vi "TFTP Get File.vi"(5 "net address":string, 6 "Binary (T)":bool=TRUE, 7 "timeout ms (1000)":i32=1000, 8 "error in (no error)":errorcluster, 9 "local path":path, 10 "remote path":string, 11 "Host":string) -> (0 "error out":errorcluster, 2 "file error":errorcluster, 3 "File Length":i32)   [LabVIEW 2016]
doc: "Connects to an TFTP server and copies a single file to the local machine."
panel:
  out "local port":u16
  out "server port":u16
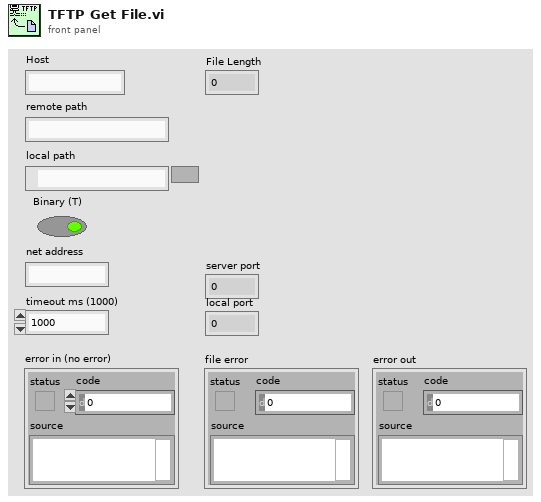
[diagram p1: front panel]
types:
  T1 = enum16{"open", "replace", "create", "open or create", "replace or create", "replace or create with confirmation"}
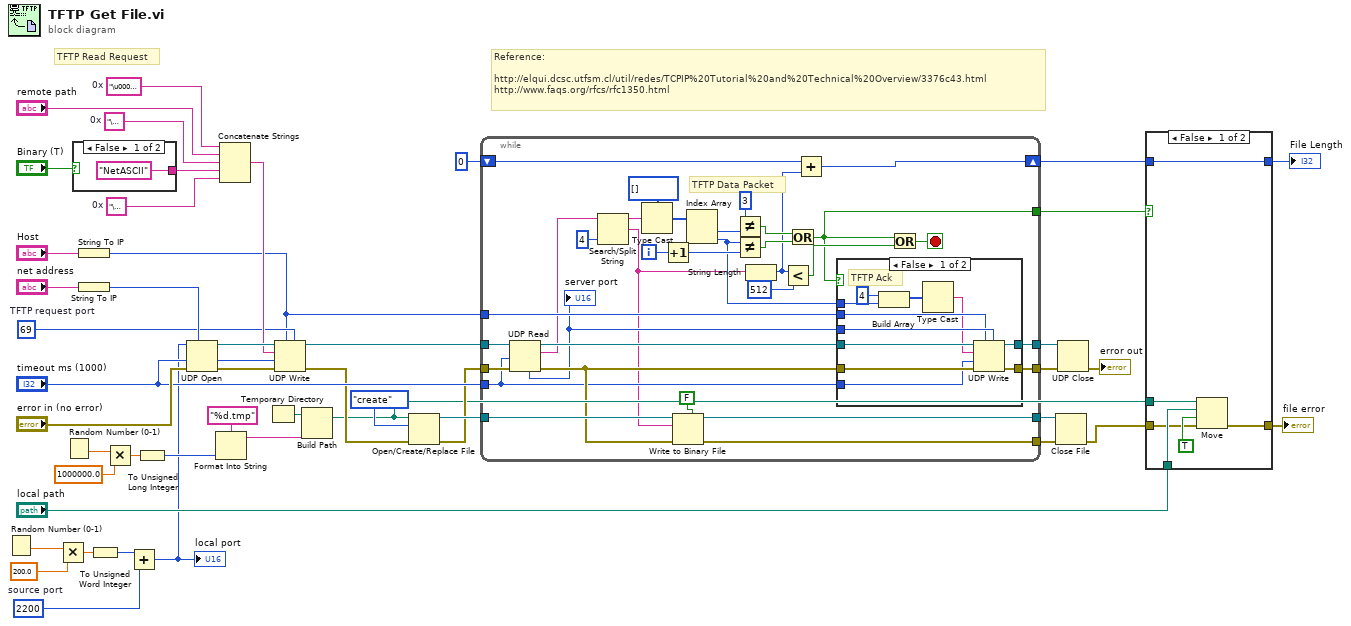
[diagram p0: block diagram]
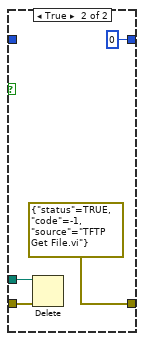
[diagram p2: hidden frame]
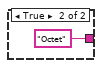
[diagram p4: hidden frame]
diagram:
  w2 = u16 2200  # source port
  w39 = "\u0000"  # 0x
  w41 = "\u0000"  # 0x
  w43 = "\u0000\u0001"  # 0x
  w34 = u16 69  # TFTP request port
  # "Reference:\n\nhttp://elqui.dcsc.utfsm.cl/util/redes/TCPIP%20Tutorial%20and%20Technical%20Overview/3376c43.html\nhttp://www.faqs.org/rfcs/rfc1350.html"
  # "TFTP Read Request"
  n1 = Random Number (0-1)() -> (number: 0 to 1=w4:dbl)
  n2 = Multiply(x=w4, y=200.0) -> (x*y=w6:dbl)
  n3 = Random Number (0-1)() -> (number: 0 to 1=w25:dbl)
  n4 = case shown="False" "Binary (T)" {
    tunnel: ["NetASCII" "Octet"] -> w40
    frame False {
    }
    frame True {
    }
  }
  n5 = String To IP(1:"Host") -> (0:w33:u32)
  n6 = String To IP(1:"net address") -> (0:w35:u32)
  n7 = To Unsigned Word Integer(number=w6) -> (unsigned 16bit integer=w3:u16)
  n8 = Multiply(x=w25, y=1000000.0) -> (x*y=w23:dbl)
  n9 = Add(x=w3, y=w2) -> (x+y=w1:u16)
  "local port" <- w1
  n10 = To Unsigned Long Integer(number=w23) -> (unsigned 32bit integer=w21:u32)
  n11 = UDP Open(7:w35, 8:"error in (no error)", 9:"timeout ms (1000)", 11:w1) -> (port=w46:refnum<k16>, 0:w45:errorcluster)  [unwired: 2 out]
  n12 = Format Into String(format string="%d.tmp", w21) -> (resulting string=w18:string)  [unwired: 2 in, 1 out]
  n13 = Concatenate Strings(w43, "remote path", w41, w40, w39) -> (w38:string)
  n14 = Temporary Directory() -> (w19:path)
  n15 = UDP Write(address=w33, port or service name=w34, connection ID=w46, data in=w38, 8:w45, 9:"timeout ms (1000)") -> (error out=w22:errorcluster, 3:w30:refnum<k16>)
  n16 = Build Path(base path=w19, name or relative path=w18) -> (appended path=w13:path)
  n17 = Open/Create/Replace File(file path (use dialog)=w13, error in=w22, operation (0:open)=T1."create") -> (refnum out=w29:refnum<file>, error out=w28:errorcluster)  [unwired: 4 out]
  n18 = while {
    tunnel: w30 -> [w82]
    tunnel: w28 -> [w81]
    tunnel: w29 -> [w70]
    tunnel: w33 -> [w64]
    tunnel: "timeout ms (1000)" -> [w62]
    tunnel: [w61] -> w27
    tunnel: [w60] -> w26
    tunnel: [w59] -> w16
    tunnel: [w58] -> w31
    tunnel: [w57] -> w15
    shift-right: [w50] -> w9
    shift-left: 0 -> [w51]
    i -> [w74]
    stop <- w67 stop-if-true
    # "TFTP Data Packet"
    n19 = UDP Read(connection ID=w82, timeout ms (25000)=w62, 8:w81) -> (data out=w56:string, error out=w65:errorcluster, 3:w66:refnum<k16>, 4:w55:u16)  [unwired: 2 out]
    "server port" <- w55
    n20 = Search/Split String(string=w56, offset (0)=4) -> (substring before match=w78:string, match + rest of string=w54:string)  [unwired: 2 out]
    n21 = Type Cast(type=u16[] [], x=w78) -> (*(type *) &x=w77:u16[])
    n22 = Increment(x=w74) -> (x+1=w73:i32)
    n23 = Write to Binary File(file (use dialog)=w70, data=w54, error in=w65, 5:FALSE ("prepend array or string size? (T)")) -> (refnum out=w61:refnum<file>, error out=w60:errorcluster)  [unwired: 3 out]
    n24 = Index Array(array=w77) -> (element #1=w76:u16, element #2=w63:u16)  [unwired: 2 in]
    n25 = Not Equal?(x=u16 3, y=w76) -> (x != y?=w71:bool)
    n26 = Not Equal?(x=w63, y=w73) -> (x != y?=w72:bool)
    n27 = String Length(string=w54) -> (length=w52:i32)
    n28 = Less?(x=w52, y=512) -> (x < y?=w68:bool)
    n29 = Or(x=w71, y=w72) -> (x .or. y?=w57:bool)
    n30 = Add(x=w51, y=w52) -> (x+y=w50:i32)
    n31 = case shown="False" w57 {
      tunnel: w66 -> [w93 w95]
      tunnel: w65 -> [w92 w94]
      tunnel: w55 -> [w91 _]
      tunnel: w64 -> [w90 _]
      tunnel: w63 -> [w88 _]
      tunnel: w62 -> [w86 _]
      tunnel: [w85 w94] -> w59
      tunnel: [w84 w95] -> w58
      frame False {
        # "TFTP Ack"
        n32 = Build Array(u16 4, w88) -> (w87:u16[])
        n33 = Type Cast(x=w87) -> (*(type *) &x=w83:string)  [unwired: 1 out]
        n34 = UDP Write(address=w90, port or service name=w91, connection ID=w93, data in=w83, 8:w92, 9:w86) -> (error out=w85:errorcluster, 3:w84:refnum<k16>)
      }
      frame True {
      }
    }
    n35 = Or(x=w57, y=w68) -> (x .or. y?=w67:bool)
  }
  n36 = Close File(refnum=w27, error in=w26) -> (error out=w12:errorcluster)  [unwired: 1 out]
  n37 = UDP Close(connection ID=w31, 8:w16) -> (error out=→"error out":errorcluster)  [unwired: 1 out]
  n38 = case shown="False" w15 {
    tunnel: "local path" -> [w99 _]
    tunnel: w13 -> [w101 w105]
    tunnel: w12 -> [w98 w104]
    tunnel: [w97 errorcluster {"status"=TRUE, "code"=-1, "source"="TFTP Get File.vi"} ("error out")] -> w11
    tunnel: w9 -> [w96 _]
    tunnel: [w96 0] -> w8
    frame False {
      n39 = Move(source path=w101, error in=w98, 9:TRUE ("overwrite (F)"), 10:w99) -> (error out=w97:errorcluster)  [unwired: 3 out]
    }
    frame True {
      n40 = Delete(path (use dialog)=w105, error in=w104) -> ()  [unwired: 6 out]
    }
  }
  "file error" <- w11
  "File Length" <- w8
